vi "WIB_Global.vi"() -> ()   [LabVIEW 2016]
uses:
  D:/share/SBND/SBND_SW/SBND_WIB_DLL/WIB_DLL/bin/Debug/WIB_DLL.dll
  SBND/SBND_SW/SBND_WIB_DLL/WIB_DLL/bin/Debug/WIB_DLL.dll
panel:
  out "WIB_DLL_REF":refnum<k24>
  out "UDP/I2C":bool=TRUE
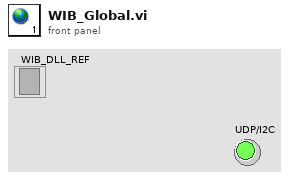
[diagram p1: front panel]
diagram:
